vi "Temperature Warnings.vi"() -> ()   [LabVIEW 2015]
panel:
  out "Warning Text":string
  out "Warning?":bool
  in  "Min temperature":dbl
  in  "Max temperature":dbl
  in  "Current Temperature":dbl
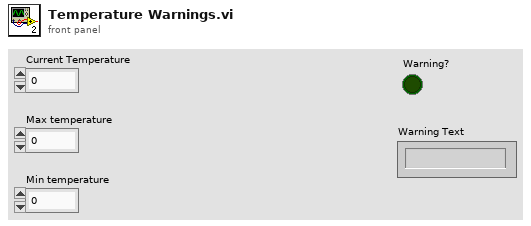
[diagram p1: front panel]
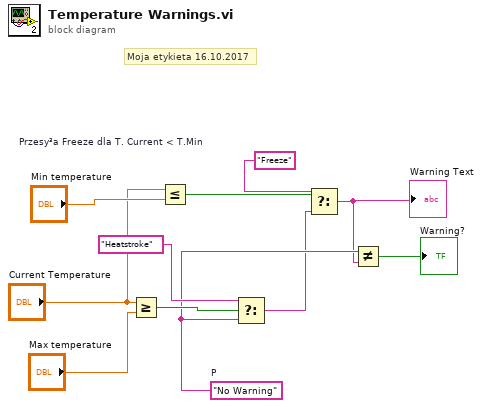
[diagram p0: block diagram]
diagram:
  w6 = "No Warning"  # P
  # "Moja etykieta 16.10.2017"
  n1 = Greater Or Equal?(x="Current Temperature", y="Max temperature") -> (x >= y?=w8:bool)
  n2 = Less Or Equal? "Przesy³a Freeze dla T. Current < T.Min"(x="Current Temperature", y="Min temperature") -> (x <= y?=w5:bool)
  n3 = Select(t="Heatstroke", s=w8, f=w6) -> (s? t:f=w3:string)
  n4 = Select(t="Freeze", s=w5, f=w3) -> (s? t:f=w1:string)
  "Warning Text" <- w1
  n5 = Not Equal?(x=w6, y=w1) -> (x != y?=→"Warning?":bool)
